vi "MAV_CMD_NAV_WAYPOINT.vi"(0 "MAVLink Waypoint":T1, 1 "Aircraft ID":u8=1) -> (4 "MAVLink Message":u8[](array[numeric]))   [LabVIEW 2014]
uses:
  Controls/MAVLink Waypoint.ctl
panel:
  out "Payload Size":i32
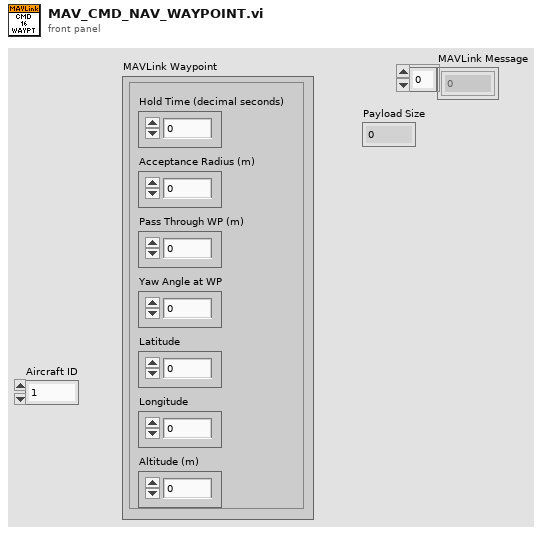
[diagram p1: front panel]
types:
  T1 = typedef "MAVLink Waypoint.ctl" = cluster{"Hold Time (decimal seconds)":sgl, "Acceptance Radius (m)":sgl, "Pass Through WP (m)":sgl, "Yaw Angle at WP":sgl, "Latitude":sgl, "Longitude":sgl, "Altitude (m)":sgl}
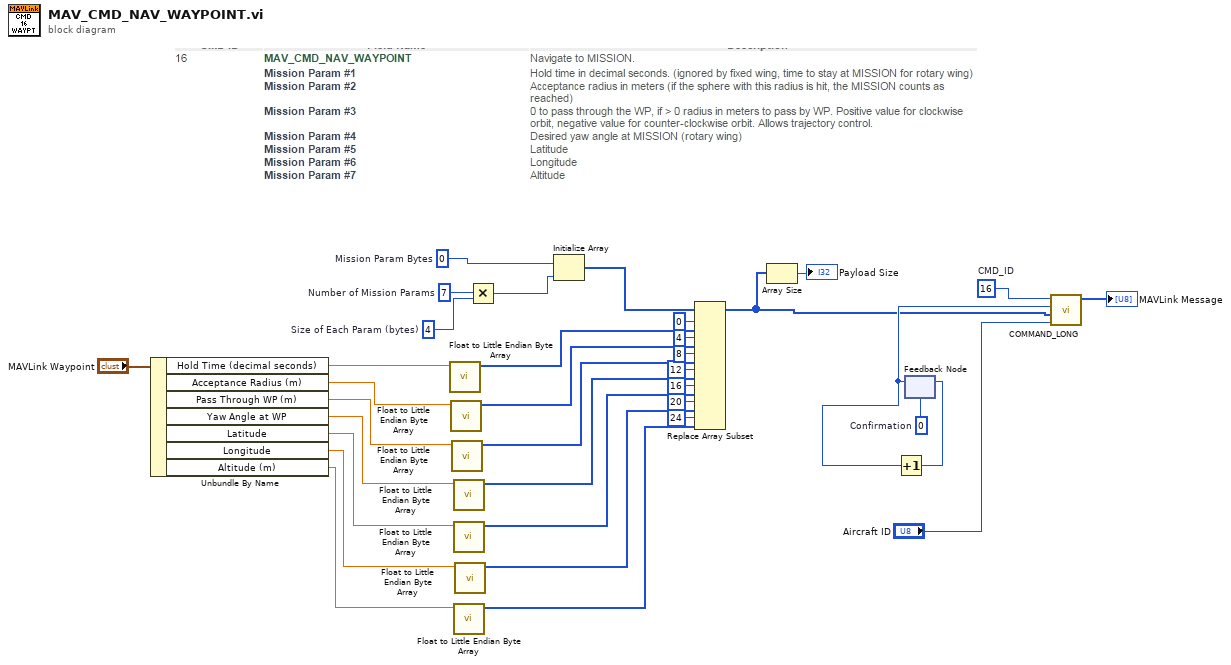
[diagram p0: block diagram]
diagram:
  w26 = u8 0  # Confirmation
  w33 = 4  # Size of Each Param (bytes)
  w34 = 7  # Number of Mission Params
  w35 = u8 0  # Mission Param Bytes
  w24 = u16 16  # CMD_ID
  n1 = Unbundle By Name("MAVLink Waypoint") -> ("Hold Time (decimal seconds)"=w7:sgl, "Acceptance Radius (m)"=w6:sgl, "Pass Through WP (m)"=w5:sgl, "Yaw Angle at WP"=w4:sgl, "Latitude"=w3:sgl, "Longitude"=w2:sgl, "Altitude (m)"=w1:sgl)
  n2 = call "Float to Little Endian Byte Array.vi"("Float In"=w7) -> ("LE Byte Array"=w20:u8[])  [unwired: 10 in]
  n3 = call "Float to Little Endian Byte Array.vi"("Float In"=w6) -> ("LE Byte Array"=w19:u8[])  [unwired: 10 in]
  n4 = call "Float to Little Endian Byte Array.vi"("Float In"=w5) -> ("LE Byte Array"=w18:u8[])  [unwired: 10 in]
  n5 = call "Float to Little Endian Byte Array.vi"("Float In"=w4) -> ("LE Byte Array"=w16:u8[])  [unwired: 10 in]
  n6 = call "Float to Little Endian Byte Array.vi"("Float In"=w3) -> ("LE Byte Array"=w14:u8[])  [unwired: 10 in]
  n7 = call "Float to Little Endian Byte Array.vi"("Float In"=w1) -> ("LE Byte Array"=w9:u8[])  [unwired: 10 in]
  n8 = call "Float to Little Endian Byte Array.vi"("Float In"=w2) -> ("LE Byte Array"=w10:u8[])  [unwired: 10 in]
  n9 = Multiply(x=w34, y=w33) -> (x*y=w32:i32)
  n10 = Initialize Array(w35, w32) -> (w31:u8[])
  n11 = Replace Array Subset(array=w31, new element #1=w20, index #1=0 ("index"), new element #2=w19, index #2=4 ("index"), new element #3=w18, index #3=8 ("index"), new element #4=w16, index #4=12 ("index"), new element #5=w14, index #5=16 ("index"), new element #6=w10, index #6=20 ("index"), new element #7=w9, index #7=24 ("index")) -> (w22:u8[])
  n12 = Array Size(array=w22) -> (size(s)=→"Payload Size":i32)
  n13 = feedback #1(w26) -> (w23:u8)
  n14 = Increment(x=w23) -> (x+1=w25:u8)
  n15 = feedback-in #1(w25) -> ()
  n16 = call "COMMAND_LONG.vi"("Target System and Target Component"="Aircraft ID", "Mission Params"=w22, "Confirmation"=w23, "Command ID"=w24) -> ("MAVLink Message"=→"MAVLink Message":u8[])  [unwired: 7 in]
